vi "FindRobotFeedbackByID.vi"(8 "error in (no error)":errorcluster, 9 "RobotsFeedback":refnum<class "RobotFeedback.lvclass">[](array[class]), 10 "id":i32, 11 "Utilities in":refnum<class "Utilities.lvclass">) -> (0 "error out":errorcluster, 1 "index":i32, 2 "RobotFeedback.lvclass":refnum<class "RobotFeedback.lvclass">, 3 "Utilities out":refnum<class "Utilities.lvclass">)   [LabVIEW 2023, in "Utilities.lvclass"]
uses:
  Utilities.lvclass
  RobotFeedback/RobotFeedback.lvclass
  RobotFeedback/RobotFeedback.lvclass/RobotFeedback.ctl
  RobotFeedback/Read id.vi
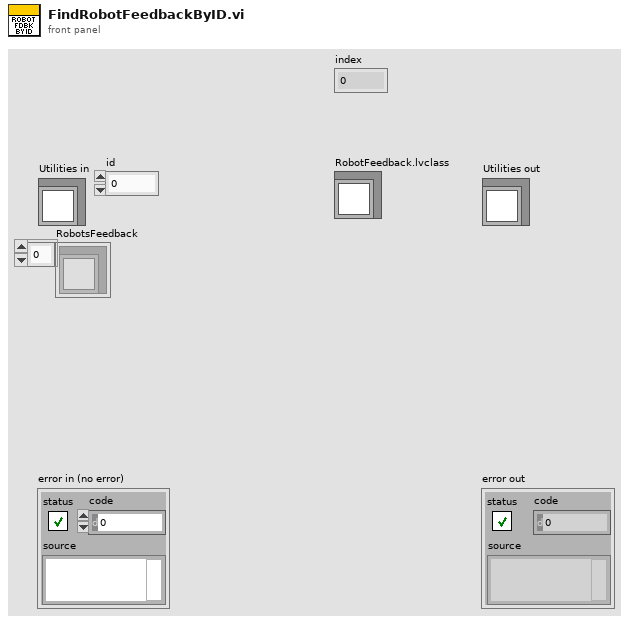
[diagram p1: front panel]
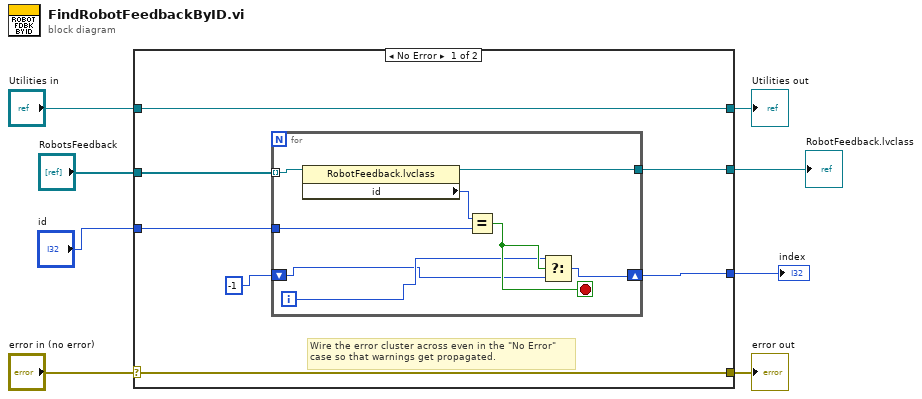
[diagram p0: block diagram]
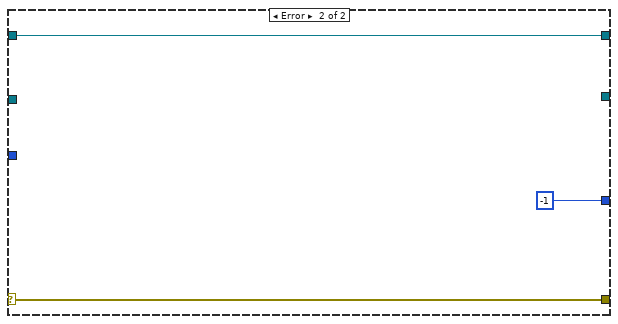
[diagram p2: hidden frame]
diagram:
  n1 = case shown="No Error" "error in (no error)" {
    selector: "error in (no error)" -> [w14 w26]
    tunnel: [w14 w26] -> w7
    tunnel: [w15 w25] -> w5
    tunnel: "Utilities in" -> [w15 w25]
    tunnel: "RobotsFeedback" -> [w13 _]
    tunnel: "id" -> [w12 _]
    tunnel: [w11 _] -> w2
    tunnel: [w10 -1] -> w1
    frame No Error {
      # "Wire the error cluster across even in the \"No Error\"\ncase so that warnings get propagated."
      n2 = for {
        tunnel: w13 -> [w23] mode=indexing
        tunnel: w12 -> [w22]
        tunnel: [w20] -> w11
        shift-right: [w17] -> w10
        shift-left: -1 -> [w16]
        i -> [w18]
        stop <- w19 stop-if-true
        n3 = property class="RobotFeedback.lvclass"(reference=w23) -> (reference out=w20:refnum<class "RobotFeedback.lvclass">, "id"=w21:i32)  [unwired: 1 in, 1 out]
        n4 = Equal?(x=w21, y=w22) -> (x = y?=w19:bool)
        n5 = Select(t=w18, s=w19, f=w16) -> (s? t:f=w17:i32)
      }
    }
    frame Error {
    }
  }
  "error out" <- w7
  "Utilities out" <- w5
  "RobotFeedback.lvclass" <- w2
  "index" <- w1
